vi "Configure.vi"(8 "error in (no error)":errorcluster, 11 "Power Meter GUI in":refnum<class "Power Meter GUI.lvclass">) -> (0 "error out":errorcluster, 3 "Power Meter GUI out":refnum<class "Power Meter GUI.lvclass">)   [LabVIEW 2020, in "Power Meter GUI.lvclass"]
doc: "Configure the measurements paramaters to sweep.\nThis should be a pop up interface invoked by the configure test button on the main panel."
uses:
  Power Meter GUI.lvclass
  Measurement.lvclass
panel:
  # "Nothing to configure"
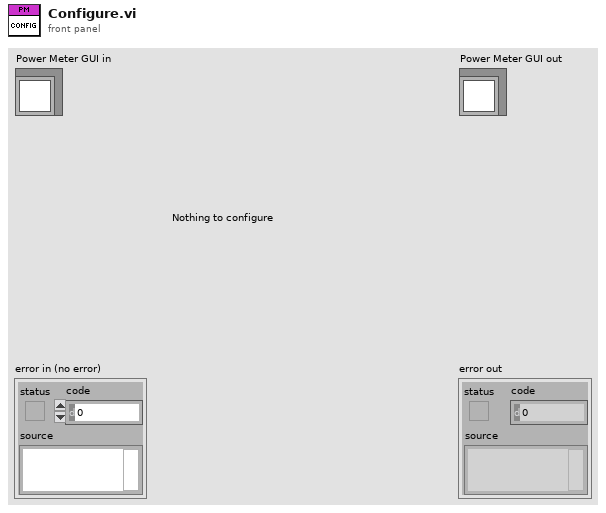
[diagram p1: front panel]
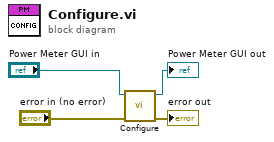
[diagram p0: block diagram]
diagram:
  n1 = call-parent "Configure.vi"("error in (no error)"="error in (no error)", "Measurements in"="Power Meter GUI in") -> ("error out"=→"error out":errorcluster, "Measurements out"=→"Power Meter GUI out":refnum<class "Power Meter GUI.lvclass">)  [unwired: 8 in]
